vi "Display Digits.vi"(7 "Digits (5 1/2)":enum16{"4 1/2", "5 1/2", "6 1/2"}(ring)=enum."5 1/2", 8 "error in":errorcluster, 9 "Channel (Channel A)":u16(ring) items=["Channel A", "Channel B"], 10 "Node In":string, 11 "VISA resource name":refnum<visa-resource-name>) -> (0 "error out":errorcluster, 2 "Node Out":string, 3 "VISA resource name out":refnum<visa-resource-name>, 4 "Command String":string)   [LabVIEW 2012, in "Keithley 2600 Series.lvlib"]
doc: "This VI sets for measurements the number of digits to display on the front panel.\n\n<b>Functions and Attributes Used</b>\ndisplay.smuX.digits"
uses:
  Keithley 2600 Series.lvlib
  Private/GlobalVariables.vi
panel:
  # "(c) 2008 Keithley Instruments, Inc.  ALL RIGHTS RESERVED."
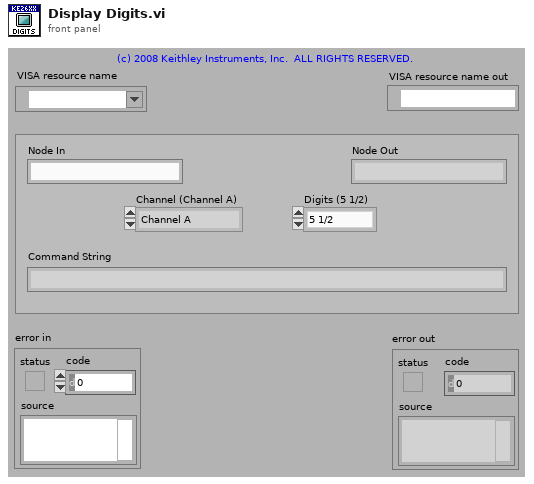
[diagram p1: front panel]
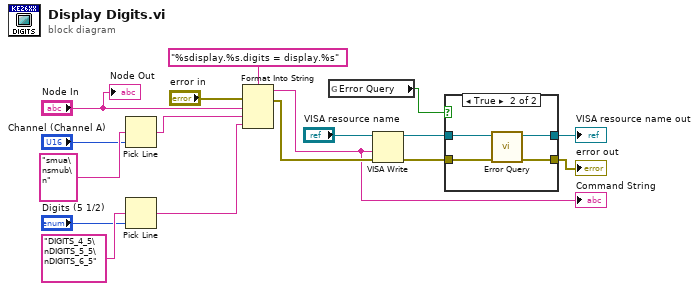
[diagram p0: block diagram]
diagram:
  n1 = Pick Line(multi-line string="smua\nsmub\n", line index="Channel (Channel A)") -> (output string=w11:string)  [unwired: 1 out]
  n2 = Pick Line(multi-line string="DIGITS_4_5\nDIGITS_5_5\nDIGITS_6_5", line index="Digits (5 1/2)") -> (output string=w10:string)  [unwired: 1 out]
  n3 = Format Into String(format string="%sdisplay.%s.digits = display.%s", error in="error in", "Node In", w11, w10) -> (resulting string=w1:string, error out=w8:errorcluster)  [unwired: 1 in]
  "Command String" <- w1
  n4 = global read "GlobalVariables.vi" "Error Query"() -> (w4:bool)
  n5 = VISA Write(VISA resource name="VISA resource name", write buffer=w1, error in (no error)=w8) -> (VISA resource name out=w6:refnum<visa-resource-name>, error out=w5:errorcluster)  [unwired: 1 out]
  n6 = case shown="True" w4 {
    tunnel: w6 -> [w19 w23]
    tunnel: w5 -> [w18 w22]
    tunnel: [w19 w21] -> w3
    tunnel: [w18 w20] -> w2
    frame False {
    }
    frame True {
      n7 = call "Error Query.vi"("error in (no error)"=w22, "VISA resource name"=w23) -> ("error out"=w20:errorcluster, "VISA resource name out"=w21:refnum<visa-resource-name>)  [unwired: 8 out]
    }
  }
  "VISA resource name out" <- w3
  "error out" <- w2
  "Node Out" <- "Node In"
